vi "RealTimeMain.vi"(6 "Header":T1, 9 "For Reference (frames)":i32=1 min=1, 11 "Motion Data":T2(array[cluster])) -> (3 "Array":dbl[][](array[numeric]))   [LabVIEW 2012]
panel:
  out "Averaging 2":bool
  in  "Col Shift Element":dbl[](array[numeric])
  in  "Vert SF":dbl[](array[numeric])
  in  "Row Shift Element":dbl[](array[numeric])
  in  "Horiz SF":dbl[](array[numeric])
  in  "Reference Frame":dbl[][][](array[numeric])
  in  "Ref Avg Count":i32
  in  "Alarm Structure":enum32{"Alarm", "Averaging"}(tab)=enum."Averaging"
  in  "Averaging":bool
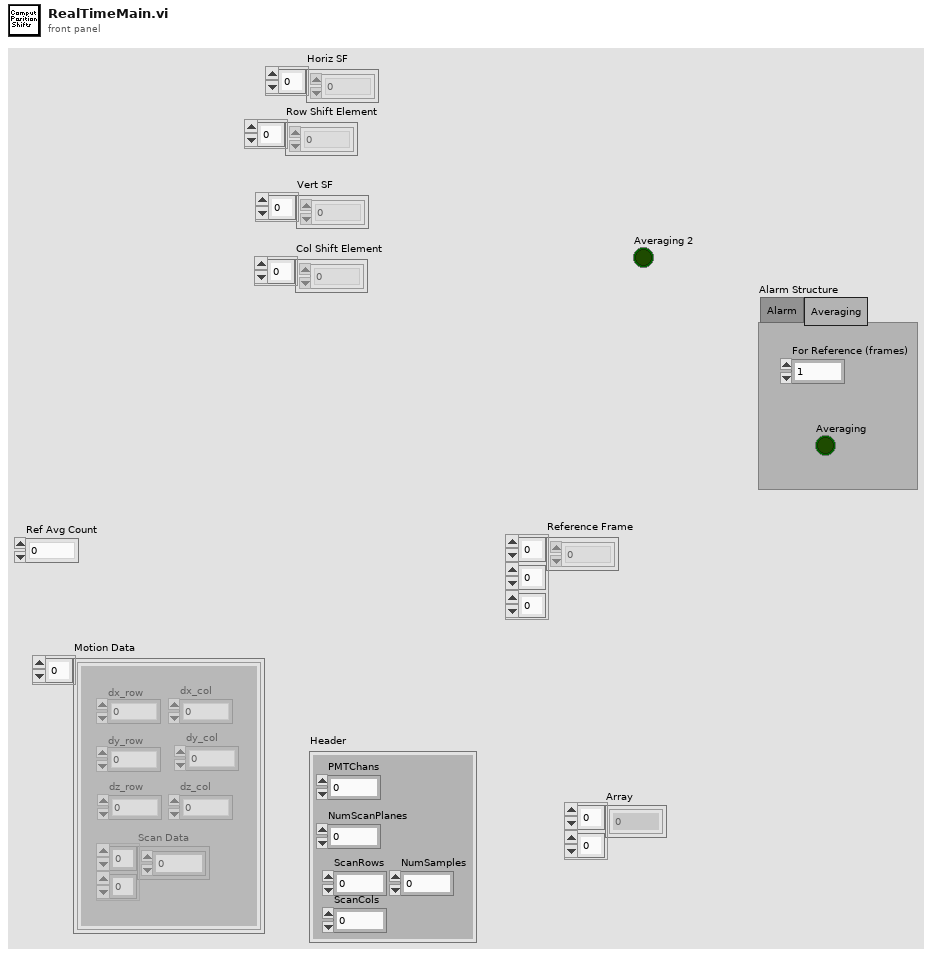
[diagram p1: front panel]
types:
  T1 = cluster{"PMTChans":i32, "NumScanPlanes":i32, "ScanRows":i32, "ScanCols":i32, "NumSamples":i32}
  T2 = cluster{"Scan Data":i32[][], "dx_row":dbl, "dy_row":dbl, "dz_row":dbl, "dx_col":dbl, "dy_col":dbl, "dz_col":dbl}[]
  T3 = cluster{"Scan Data":i32[][], "dx_row":dbl, "dy_row":dbl, "dz_row":dbl, "dx_col":dbl, "dy_col":dbl, "dz_col":dbl}
  T4 = cluster{"dx_row":dbl, "dy_row":dbl, "dz_row":dbl, "dx_col":dbl, "dy_col":dbl, "dz_col":dbl}
  T5 = cluster{"X1":dbl[], "Y1":dbl[], "Z1":dbl[], "X2":dbl[], "Y2":dbl[], "Z2":dbl[]}
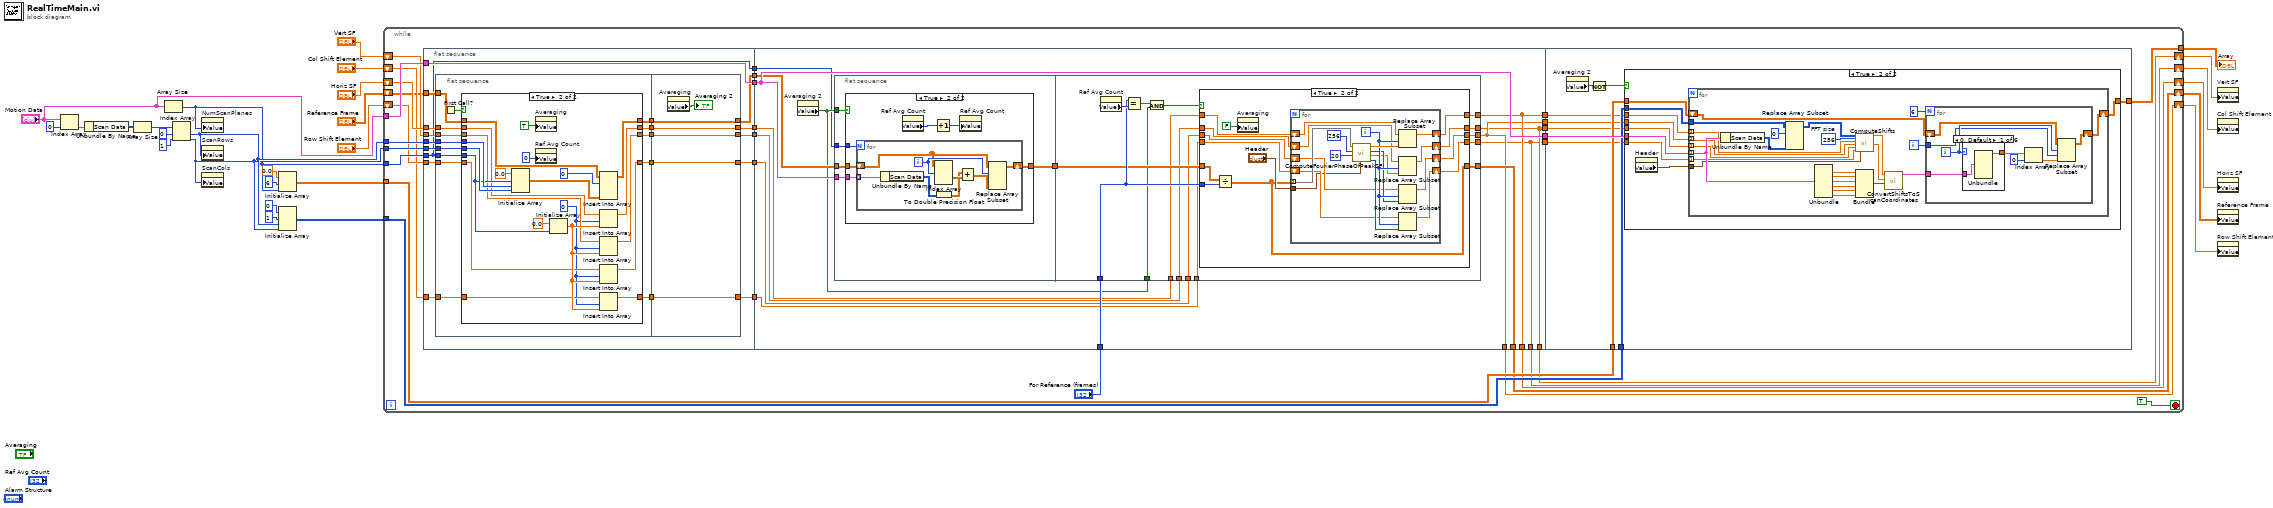
[diagram p0: block diagram]
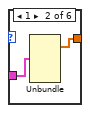
[diagram p6: hidden frame]
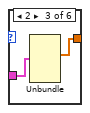
[diagram p7: hidden frame]
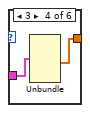
[diagram p8: hidden frame]
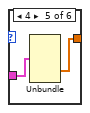
[diagram p9: hidden frame]
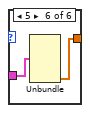
[diagram p10: hidden frame]
diagram:
  n1 = Index Array(array="Motion Data", index=0) -> (element=w26:T3)
  n2 = Unbundle By Name(w26) -> ("Scan Data"=w25:i32[][])
  n3 = Array Size(array=w25) -> (size(s)=w24:i32[])
  n4 = Array Size(array="Motion Data") -> (size(s)=w14:i32)
  n5 = Index Array(array=w24, index #1=0 ("index"), index #2=1 ("index")) -> (element #1=w17:i32, element #2=w16:i32)
  n6 = property on="NumScanPlanes" class="DigNum (strict)"("Value"=w14) -> ()  [unwired: 2 in, 2 out]
  n7 = property on="ScanRows" class="DigNum (strict)"("Value"=w17) -> ()  [unwired: 2 in, 2 out]
  n8 = property on="ScanCols" class="DigNum (strict)"("Value"=w16) -> ()  [unwired: 2 in, 2 out]
  n9 = Initialize Array(0.0 ("element"), 6 ("dimension size"), w14) -> (w12:dbl[][])
  n10 = Initialize Array(0 ("element"), 1 ("dimension size"), w17, w16) -> (w18:i32[][][])
  n11 = while {
    tunnel: "Motion Data" -> [w47]
    tunnel: w18 -> [w45]
    tunnel: w17 -> [w44]
    tunnel: w16 -> [w43]
    tunnel: w14 -> [w42]
    tunnel: w12 -> [w41]
    shift-right: [w35] -> w6
    shift-left: "Reference Frame" -> [w28]
    tunnel: [w36] -> w1
    shift-right: [w34] -> w5
    shift-left: "Horiz SF" -> [w40]
    shift-right: [w33] -> w4
    shift-left: "Row Shift Element" -> [w39]
    shift-right: [w32] -> w3
    shift-left: "Vert SF" -> [w38]
    shift-right: [w31] -> w2
    shift-left: "Col Shift Element" -> [w37]
    stop <- TRUE stop-if-true
    n12 = flat-sequence {
      tunnel: w47 -> [w77]
      tunnel: [w77] -> w58
      tunnel: w42 -> [w59]
      tunnel: w44 -> [w76]
      tunnel: w43 -> [w60]
      tunnel: w28 -> [w75]
      tunnel: [w74] -> w57
      tunnel: w40 -> [w73]
      tunnel: w39 -> [w72]
      tunnel: w38 -> [w71]
      tunnel: w37 -> [w70]
      tunnel: [w69] -> w56
      tunnel: [w68] -> w55
      tunnel: [w67] -> w54
      tunnel: [w66] -> w53
      tunnel: [w59] -> w30
      tunnel: w58 -> [w136]
      tunnel: "For Reference (frames)" -> [w138]
      tunnel: [w136] -> w52
      tunnel: w57 -> [w135]
      tunnel: w56 -> [w134]
      tunnel: w55 -> [w133]
      tunnel: w54 -> [w132]
      tunnel: w53 -> [w131]
      tunnel: [w128] -> w51
      tunnel: [w127] -> w50
      tunnel: [w126] -> w49
      tunnel: [w125] -> w48
      tunnel: [w129] -> w35
      tunnel: [w128] -> w34
      tunnel: [w127] -> w33
      tunnel: [w126] -> w32
      tunnel: [w125] -> w31
      tunnel: w30 -> [w124]
      tunnel: w52 -> [w218]
      tunnel: w45 -> [w217]
      tunnel: w41 -> [w216]
      tunnel: w51 -> [w215]
      tunnel: w50 -> [w214]
      tunnel: w49 -> [w213]
      tunnel: w48 -> [w212]
      tunnel: [w211] -> w36
      frame #0 {
        n13 = flat-sequence {
          tunnel: w59 -> [w91]
          tunnel: w76 -> [w90]
          tunnel: w60 -> [w89]
          tunnel: w75 -> [w88]
          tunnel: w73 -> [w86]
          tunnel: w72 -> [w85]
          tunnel: w71 -> [w84]
          tunnel: w70 -> [w83]
          tunnel: [w87] -> w65
          tunnel: [w82] -> w64
          tunnel: [w81] -> w63
          tunnel: [w80] -> w62
          tunnel: [w79] -> w61
          tunnel: [w119] -> w66
          tunnel: [w120] -> w67
          tunnel: [w121] -> w68
          tunnel: [w122] -> w69
          tunnel: [w123] -> w74
          tunnel: w65 -> [w123]
          tunnel: w64 -> [w122]
          tunnel: w63 -> [w121]
          tunnel: w62 -> [w120]
          tunnel: w61 -> [w119]
          frame #0 {
            n14 = First Call?() -> (First Call?: T/F=w78:bool)
            n15 = case shown="True" w78 {
              tunnel: w91 -> [_ w109]
              tunnel: w90 -> [_ w116]
              tunnel: w89 -> [_ w115]
              tunnel: w88 -> [w96 w114]
              tunnel: [w96 w112] -> w87
              tunnel: w86 -> [w94 w108]
              tunnel: w85 -> [w93 w106]
              tunnel: w84 -> [w95 w105]
              tunnel: w83 -> [w92 w104]
              tunnel: [w94 w102] -> w82
              tunnel: [w93 w101] -> w81
              tunnel: [w95 w100] -> w80
              tunnel: [w92 w99] -> w79
              frame False {
              }
              frame True {
                w97 = 0 ("index")
                n16 = Initialize Array(0.0 ("element"), w109, w116, w115) -> (w113:dbl[][][])
                n17 = property on="Averaging" class="Bool (strict)"("Value"=TRUE) -> ()  [unwired: 2 in, 2 out]
                n18 = property on="Ref Avg Count" class="DigNum (strict)"("Value"=0 ("Ref Avg Count")) -> ()  [unwired: 2 in, 2 out]
                n19 = Initialize Array(0.0 ("element"), w109) -> (w107:dbl[])
                n20 = Insert Into Array(array=w114, index (dim 0)=0 ("index (page)"), new element=w113) -> (w112:dbl[][][])  [unwired: 2 in]
                n21 = Insert Into Array(array=w108, index=w97, new element=w107) -> (w102:dbl[])
                n22 = Insert Into Array(array=w105, index=w97, new element=w107) -> (w100:dbl[])
                n23 = Insert Into Array(array=w106, index=w97, new element=w107) -> (w101:dbl[])
                n24 = Insert Into Array(array=w104, index=w97, new element=w107) -> (w99:dbl[])
              }
            }
          }
          frame #1 {
            n25 = property on="Averaging" class="Bool (strict)"() -> ("Value"=→"Averaging 2":bool)  [unwired: 2 in, 2 out]
          }
        }
      }
      frame #1 {
        n26 = property on="Averaging 2" class="Bool (strict)"() -> ("Value"=w130:bool)  [unwired: 2 in, 2 out]
        n27 = flat-sequence {
          tunnel: w136 -> [w143]
          tunnel: w130 -> [w142]
          tunnel: [w141] -> w137
          tunnel: w135 -> [w140]
          tunnel: w124 -> [w139]
          tunnel: w138 -> [w170]
          tunnel: w137 -> [w169]
          tunnel: w134 -> [w168]
          tunnel: w133 -> [w167]
          tunnel: w132 -> [w166]
          tunnel: w131 -> [w165]
          tunnel: [w164] -> w128
          tunnel: [w163] -> w127
          tunnel: [w162] -> w126
          tunnel: [w161] -> w125
          tunnel: w130 -> [w160]
          tunnel: [w159] -> w129
          frame #0 {
            n28 = case shown="True" w142 {
              tunnel: w143 -> [_ w150]
              tunnel: [w144 w149] -> w141
              tunnel: w140 -> [w144 w148]
              tunnel: w139 -> [_ w145]
              frame False {
              }
              frame True {
                n29 = for {
                  N: w145 -> [_]
                  tunnel: w150 -> [w158] mode=indexing
                  shift-right: [w153] -> w149
                  shift-left: w148 -> [w155]
                  i -> [w156]
                  n30 = Unbundle By Name(w158) -> ("Scan Data"=w152:i32[][])
                  n31 = Index Array(array=w155, index (dim 0)=w156) -> (element=w157:dbl[][])  [unwired: 2 in]
                  n32 = To Double Precision Float(number=w152) -> (double precision float=w151:dbl[][])
                  n33 = Add(x=w151, y=w157) -> (x+y=w154:dbl[][])
                  n34 = Replace Array Subset(array=w155, new element=w154, index (dim 0)=w156) -> (w153:dbl[][][])  [unwired: 2 in]
                }
                n35 = property on="Ref Avg Count" class="DigNum (strict)"() -> ("Value"=w147:i32)  [unwired: 2 in, 2 out]
                n36 = Increment(x=w147) -> (x+1=w146:i32)
                n37 = property on="Ref Avg Count" class="DigNum (strict)"("Value"=w146) -> ()  [unwired: 2 in, 2 out]
              }
            }
          }
          frame #1 {
            n38 = property on="Ref Avg Count" class="DigNum (strict)"() -> ("Value"=w171:i32)  [unwired: 2 in, 2 out]
            n39 = Equal?(x=w170, y=w171) -> (x = y?=w173:bool)
            n40 = And(x=w173, y=w160) -> (x .and. y?=w172:bool)
            n41 = case shown="True" w172 {
              tunnel: w169 -> [w174 w191]
              tunnel: w170 -> [_ w190]
              tunnel: w168 -> [w175 w189]
              tunnel: w167 -> [w176 w188]
              tunnel: w166 -> [w177 w187]
              tunnel: w165 -> [w178 w186]
              tunnel: [w175 w185] -> w164
              tunnel: [w176 w184] -> w163
              tunnel: [w177 w183] -> w162
              tunnel: [w178 w182] -> w161
              tunnel: [w174 w179] -> w159
              frame False {
              }
              frame True {
                n42 = Divide(x=w191, y=w190) -> (x/y=w179:dbl[][][])
                n43 = property on="Averaging" class="Bool (strict)"("Value"=FALSE) -> ()  [unwired: 2 in, 2 out]
                n44 = for {
                  tunnel: w179 -> [w208] mode=indexing
                  shift-right: [w196] -> w185
                  shift-left: w189 -> [w200]
                  shift-right: [w195] -> w184
                  shift-left: w188 -> [w199]
                  shift-right: [w194] -> w183
                  shift-left: w187 -> [w198]
                  shift-right: [w193] -> w182
                  shift-left: w186 -> [w197]
                  tunnel: "Header" -> [w192]
                  i -> [w204]
                  n45 = call "ComputeFourierPhaseOfPeakSF.vi"("Header"=w192, "Search SF Limit"=20, "FFT size"=256, "Scan Frame"=w208) -> ("Col Shift Element Number"=w201:i32, "Vertical SF Phase"=w202:dbl, "Row Shift Element Numbert"=w203:i32, "Horizontal SF Phase"=w205:dbl)  [unwired: 4 in]
                  n46 = Replace Array Subset(array=w200, new element=w205, index=w204) -> (w196:dbl[])
                  n47 = Replace Array Subset(array=w198, new element=w202, index=w204) -> (w194:dbl[])
                  n48 = Replace Array Subset(array=w199, new element=w203, index=w204) -> (w195:dbl[])
                  n49 = Replace Array Subset(array=w197, new element=w201, index=w204) -> (w193:dbl[])
                }
              }
            }
          }
        }
      }
      frame #2 {
        n50 = property on="Averaging 2" class="Bool (strict)"() -> ("Value"=w210:bool)  [unwired: 2 in, 2 out]
        n51 = Not(x=w210) -> (.not. x?=w209:bool)
        n52 = case shown="True" w209 {
          tunnel: w218 -> [_ w228]
          tunnel: w217 -> [_ w227]
          tunnel: [w219 w226] -> w211
          tunnel: w216 -> [w219 w225]
          tunnel: w215 -> [_ w224]
          tunnel: w214 -> [_ w223]
          tunnel: w213 -> [_ w222]
          tunnel: w212 -> [_ w221]
          frame False {
          }
          frame True {
            n53 = property on="Header" class="Clust (strict)"() -> ("Value"=w220:T1)  [unwired: 2 in, 2 out]
            n54 = for {
              tunnel: w228 -> [w246] mode=indexing
              tunnel: w227 -> [w250]
              tunnel: w220 -> [w238]
              shift-right: [w236] -> w226
              shift-left: w225 -> [w237]
              tunnel: w224 -> [w232] mode=indexing
              tunnel: w223 -> [w231] mode=indexing
              tunnel: w222 -> [w230] mode=indexing
              tunnel: w221 -> [w229] mode=indexing
              i -> [w235]
              w253 = 256  # FFT size
              n55 = Unbundle By Name(w246) -> ("Scan Data"=w248:i32[][])
              n56 = Replace Array Subset(array=w250, new element=w248, index (dim 0)=0 ("index (row)")) -> (w247:i32[][][])  [unwired: 2 in]
              n57 = Unbundle(w246) -> ("dx_row"=w245:dbl, "dy_row"=w244:dbl, "dz_row"=w243:dbl, "dx_col"=w242:dbl, "dy_col"=w241:dbl, "dz_col"=w240:dbl)  [unwired: 1 out]
              n58 = call "ComputeShifts.vi"("Scan Plane Data"=w247, "FFT size"=w253, "Ref Horizontal SF Phase"=w232, "Ref Row Shift Element"=w231, "Ref Vertical SF Phase"=w230, "Ref Col Shift Element"=w229, "Header"=w238) -> ("Row Shift Array"=w252:dbl[], "Col Shift Array"=w251:dbl[])  [unwired: 11 in]
              n59 = Bundle("dx_row"=w245, "dy_row"=w244, "dz_row"=w243, "dx_col"=w242, "dy_col"=w241, "dz_col"=w240) -> (w239:T4)  [unwired: 1 in]
              n60 = call "ConvertShiftsToScanCoordinates.vi"("PixelToScanCoordConvFactors"=w239, "Col Shift Array"=w251, "Row Shift Array"=w252) -> ("Motion"=w234:T5)  [unwired: 8 in]
              n61 = for {
                N: 6 -> [_]
                shift-right: [w254] -> w236
                shift-left: w237 -> [w257]
                tunnel: w235 -> [w255]
                tunnel: w234 -> [w261]
                i -> [w256]
                n62 = case shown="0, Default" w256 {
                  tunnel: [w262 w264 w266 w268 w270 w272] -> w260
                  tunnel: w261 -> [w263 w265 w267 w269 w271 w273]
                  frame 0, Default {
                    n63 = Unbundle(w263) -> ("X1"=w262:dbl[])  [unwired: 5 out]
                  }
                  frame 1 {
                    n64 = Unbundle(w265) -> ("Y1"=w264:dbl[])  [unwired: 5 out]
                  }
                  frame 2 {
                    n65 = Unbundle(w267) -> ("Z1"=w266:dbl[])  [unwired: 5 out]
                  }
                  frame 3 {
                    n66 = Unbundle(w269) -> ("X2"=w268:dbl[])  [unwired: 5 out]
                  }
                  frame 4 {
                    n67 = Unbundle(w271) -> ("Y2"=w270:dbl[])  [unwired: 5 out]
                  }
                  frame 5 {
                    n68 = Unbundle(w273) -> ("Z2"=w272:dbl[])  [unwired: 5 out]
                  }
                }
                n69 = Index Array(array=w260, index=0) -> (element=w258:dbl)
                n70 = Replace Array Subset(array=w257, new element=w258, index (row)=w256, index (col)=w255) -> (w254:dbl[][])
              }
            }
          }
        }
      }
    }
  }
  "Array" <- w1
  n71 = property on="Vert SF" class="Arr (strict)"("Value"=w3) -> ()  [unwired: 2 in, 2 out]
  n72 = property on="Col Shift Element" class="Arr (strict)"("Value"=w2) -> ()  [unwired: 2 in, 2 out]
  n73 = property on="Horiz SF" class="Arr (strict)"("Value"=w5) -> ()  [unwired: 2 in, 2 out]
  n74 = property on="Reference Frame" class="Arr (strict)"("Value"=w6) -> ()  [unwired: 2 in, 2 out]
  n75 = property on="Row Shift Element" class="Arr (strict)"("Value"=w4) -> ()  [unwired: 2 in, 2 out]
